vi "cast_dw_to_32_bit.vi"(8 "input valid":bool=TRUE, 10 "Shift":i32, 11 "x":fxp<+/-,64,48>) -> (0 "output valid":bool, 3 "y":fxp<+/-,32,14>)   [LabVIEW 2018]
uses:
  <vilib>/rvi/FXPMathLib/FxpConvert/subVIs/nifxpmath_Convert_SimConfig.ctl
  <vilib>/fxp/LVFixedPointQuantizationPolicyTypeDef.ctl
  <vilib>/fxp/LVFixedPointOverflowPolicyTypeDef.ctl
  <vilib>/rvi/FXPMathLib/FxpConvert/simVIs/DllFxpConvertTemp_sub.vi
  <vilib>/rvi/FXPMathLib/FxpInterpret/XNode/nifxpmath_Interpret.xnode
  <vilib>/rvi/FXPMathLib/FxpConvert/XNode/nifxpmath_Convert.xnode
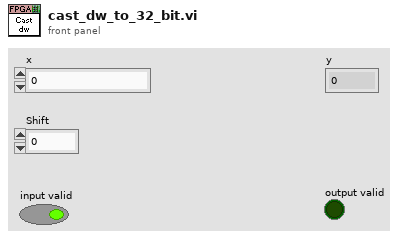
[diagram p1: front panel]
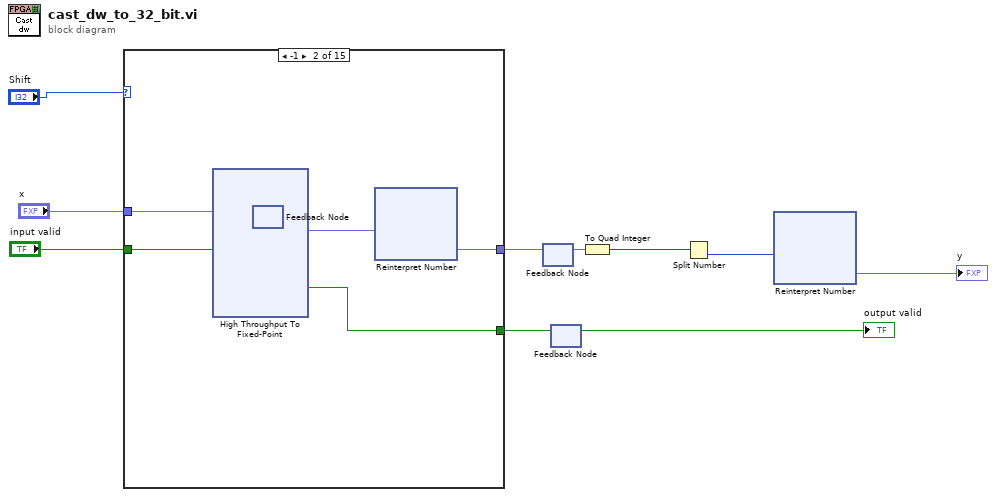
[diagram p0: block diagram]
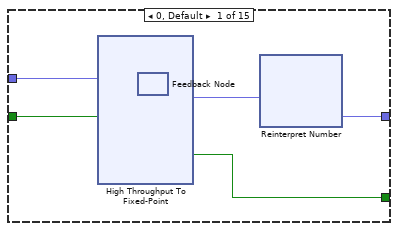
[diagram p2: hidden frame]
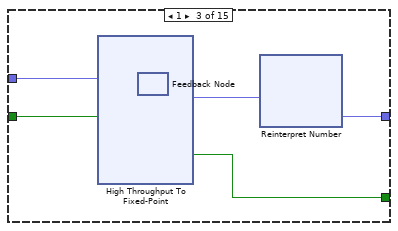
[diagram p3: hidden frame]
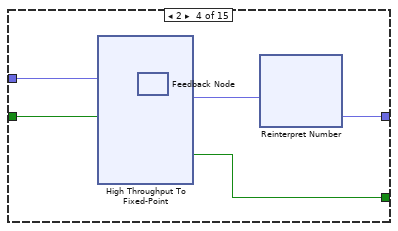
[diagram p4: hidden frame]
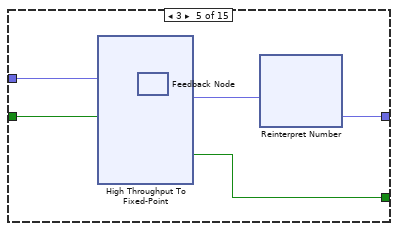
[diagram p5: hidden frame]
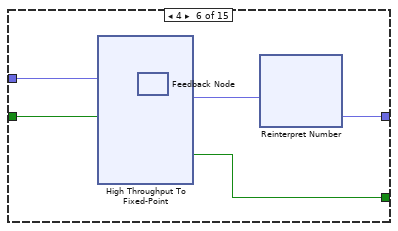
[diagram p6: hidden frame]
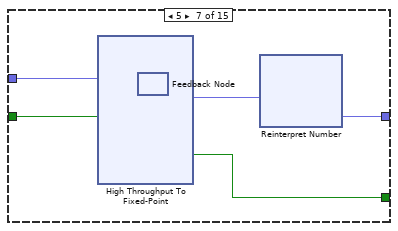
[diagram p7: hidden frame]
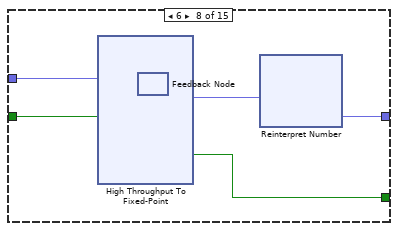
[diagram p8: hidden frame]
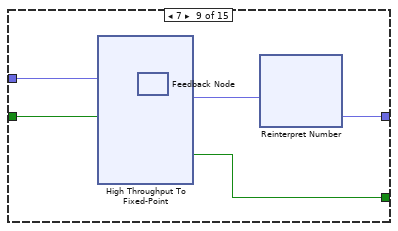
[diagram p9: hidden frame]
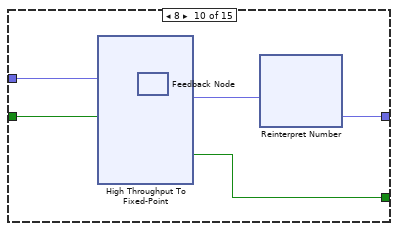
[diagram p10: hidden frame]
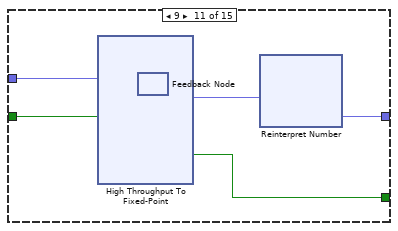
[diagram p11: hidden frame]
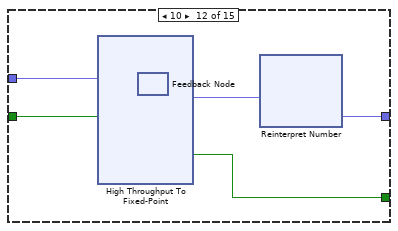
[diagram p12: hidden frame]
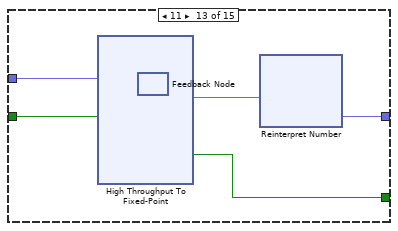
[diagram p13: hidden frame]
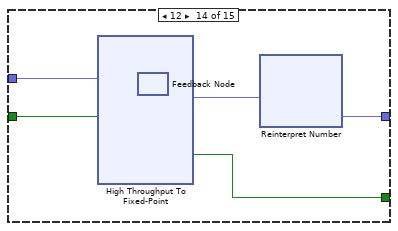
[diagram p14: hidden frame]
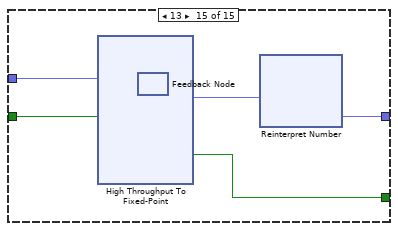
[diagram p15: hidden frame]
diagram:
  n1 = case shown="-1" "Shift" {
    tunnel: [w15 w44 w73 w102 w131 w160 w189 w218 w247 w276 w305 w334 w363 w392 w421] -> w9
    tunnel: "x" -> [w14 w43 w72 w101 w130 w159 w188 w217 w246 w275 w304 w333 w362 w391 w420]
    tunnel: "input valid" -> [w13 w42 w71 w100 w129 w158 w187 w216 w245 w274 w303 w332 w361 w390 w419]
    tunnel: [w12 w41 w70 w99 w128 w157 w186 w215 w244 w273 w302 w331 w360 w389 w418] -> w2
    frame 0, Default {
      n2 = xnode "High Throughput To Fixed-Point"("x"=w14, "input valid"=w13) -> ("y"=w11:fxp<+/-,64,46>, "output valid"=w12:bool)  [unwired: 1 in, 1 out]
      n3 = feedback #1() -> ()  [unwired: 2 in]
      n4 = feedback-in #1(w14) -> ()
      n5 = xnode "Reinterpret Number"("x"=w11) -> ("y"=w15:fxp<+/-,64,64>)
    }
    frame -1 {
      n6 = xnode "High Throughput To Fixed-Point"("x"=w43, "input valid"=w42) -> ("y"=w40:fxp<+/-,64,45>, "output valid"=w41:bool)  [unwired: 1 in, 1 out]
      n7 = feedback #2() -> ()  [unwired: 2 in]
      n8 = feedback-in #2(w43) -> ()
      n9 = xnode "Reinterpret Number"("x"=w40) -> ("y"=w44:fxp<+/-,64,64>)
    }
    frame 1 {
      n10 = xnode "High Throughput To Fixed-Point"("x"=w72, "input valid"=w71) -> ("y"=w69:fxp<+/-,64,47>, "output valid"=w70:bool)  [unwired: 1 in, 1 out]
      n11 = feedback #3() -> ()  [unwired: 2 in]
      n12 = feedback-in #3(w72) -> ()
      n13 = xnode "Reinterpret Number"("x"=w69) -> ("y"=w73:fxp<+/-,64,64>)
    }
    frame 2 {
      n14 = xnode "High Throughput To Fixed-Point"("x"=w101, "input valid"=w100) -> ("y"=w98:fxp<+/-,64,48>, "output valid"=w99:bool)  [unwired: 1 in, 1 out]
      n15 = feedback #4() -> ()  [unwired: 2 in]
      n16 = feedback-in #4(w101) -> ()
      n17 = xnode "Reinterpret Number"("x"=w98) -> ("y"=w102:fxp<+/-,64,64>)
    }
    frame 3 {
      n18 = xnode "High Throughput To Fixed-Point"("x"=w130, "input valid"=w129) -> ("y"=w127:fxp<+/-,64,49>, "output valid"=w128:bool)  [unwired: 1 in, 1 out]
      n19 = feedback #5() -> ()  [unwired: 2 in]
      n20 = feedback-in #5(w130) -> ()
      n21 = xnode "Reinterpret Number"("x"=w127) -> ("y"=w131:fxp<+/-,64,64>)
    }
    frame 4 {
      n22 = xnode "High Throughput To Fixed-Point"("x"=w159, "input valid"=w158) -> ("y"=w156:fxp<+/-,64,50>, "output valid"=w157:bool)  [unwired: 1 in, 1 out]
      n23 = feedback #6() -> ()  [unwired: 2 in]
      n24 = feedback-in #6(w159) -> ()
      n25 = xnode "Reinterpret Number"("x"=w156) -> ("y"=w160:fxp<+/-,64,64>)
    }
    frame 5 {
      n26 = xnode "High Throughput To Fixed-Point"("x"=w188, "input valid"=w187) -> ("y"=w185:fxp<+/-,64,51>, "output valid"=w186:bool)  [unwired: 1 in, 1 out]
      n27 = feedback #7() -> ()  [unwired: 2 in]
      n28 = feedback-in #7(w188) -> ()
      n29 = xnode "Reinterpret Number"("x"=w185) -> ("y"=w189:fxp<+/-,64,64>)
    }
    frame 6 {
      n30 = xnode "High Throughput To Fixed-Point"("x"=w217, "input valid"=w216) -> ("y"=w214:fxp<+/-,64,52>, "output valid"=w215:bool)  [unwired: 1 in, 1 out]
      n31 = feedback #8() -> ()  [unwired: 2 in]
      n32 = feedback-in #8(w217) -> ()
      n33 = xnode "Reinterpret Number"("x"=w214) -> ("y"=w218:fxp<+/-,64,64>)
    }
    frame 7 {
      n34 = xnode "High Throughput To Fixed-Point"("x"=w246, "input valid"=w245) -> ("y"=w243:fxp<+/-,64,53>, "output valid"=w244:bool)  [unwired: 1 in, 1 out]
      n35 = feedback #9() -> ()  [unwired: 2 in]
      n36 = feedback-in #9(w246) -> ()
      n37 = xnode "Reinterpret Number"("x"=w243) -> ("y"=w247:fxp<+/-,64,64>)
    }
    frame 8 {
      n38 = xnode "High Throughput To Fixed-Point"("x"=w275, "input valid"=w274) -> ("y"=w272:fxp<+/-,64,54>, "output valid"=w273:bool)  [unwired: 1 in, 1 out]
      n39 = feedback #10() -> ()  [unwired: 2 in]
      n40 = feedback-in #10(w275) -> ()
      n41 = xnode "Reinterpret Number"("x"=w272) -> ("y"=w276:fxp<+/-,64,64>)
    }
    frame 9 {
      n42 = xnode "High Throughput To Fixed-Point"("x"=w304, "input valid"=w303) -> ("y"=w301:fxp<+/-,64,55>, "output valid"=w302:bool)  [unwired: 1 in, 1 out]
      n43 = feedback #11() -> ()  [unwired: 2 in]
      n44 = feedback-in #11(w304) -> ()
      n45 = xnode "Reinterpret Number"("x"=w301) -> ("y"=w305:fxp<+/-,64,64>)
    }
    frame 10 {
      n46 = xnode "High Throughput To Fixed-Point"("x"=w333, "input valid"=w332) -> ("y"=w330:fxp<+/-,64,56>, "output valid"=w331:bool)  [unwired: 1 in, 1 out]
      n47 = feedback #12() -> ()  [unwired: 2 in]
      n48 = feedback-in #12(w333) -> ()
      n49 = xnode "Reinterpret Number"("x"=w330) -> ("y"=w334:fxp<+/-,64,64>)
    }
    frame 11 {
      n50 = xnode "High Throughput To Fixed-Point"("x"=w362, "input valid"=w361) -> ("y"=w359:fxp<+/-,64,57>, "output valid"=w360:bool)  [unwired: 1 in, 1 out]
      n51 = feedback #13() -> ()  [unwired: 2 in]
      n52 = feedback-in #13(w362) -> ()
      n53 = xnode "Reinterpret Number"("x"=w359) -> ("y"=w363:fxp<+/-,64,64>)
    }
    frame 12 {
      n54 = xnode "High Throughput To Fixed-Point"("x"=w391, "input valid"=w390) -> ("y"=w388:fxp<+/-,64,58>, "output valid"=w389:bool)  [unwired: 1 in, 1 out]
      n55 = feedback #14() -> ()  [unwired: 2 in]
      n56 = feedback-in #14(w391) -> ()
      n57 = xnode "Reinterpret Number"("x"=w388) -> ("y"=w392:fxp<+/-,64,64>)
    }
    frame 13 {
      n58 = xnode "High Throughput To Fixed-Point"("x"=w420, "input valid"=w419) -> ("y"=w417:fxp<+/-,64,59>, "output valid"=w418:bool)  [unwired: 1 in, 1 out]
      n59 = feedback #15() -> ()  [unwired: 2 in]
      n60 = feedback-in #15(w420) -> ()
      n61 = xnode "Reinterpret Number"("x"=w417) -> ("y"=w421:fxp<+/-,64,64>)
    }
  }
  n62 = feedback #16() -> (w6:fxp<+/-,64,64>)  [unwired: 1 in]
  n63 = feedback-in #16(w9) -> ()
  n64 = feedback #17() -> (→"output valid":bool)  [unwired: 1 in]
  n65 = feedback-in #17(w2) -> ()
  n66 = To Quad Integer(1:w6) -> (0:w10:i64)
  n67 = Split Number(x=w10) -> (lo(x)=w8:u32)  [unwired: 1 out]
  n68 = xnode "Reinterpret Number"("x"=w8) -> ("y"=→"y":fxp<+/-,32,14>)
